vi "sequencerCycleLoops.vi"(6 "kepcoScan":bool, 8 "nOfCycles":i32 format="%0d", 9 "nOfLoops":i32 format="%0d", 11 "Array of Tracks":i32[](array[numeric])=[0, 0, 0, 0, 0, 0, 0, 0, 0, 0, 0, 0, 0, 0, 0, 0, 0, 0, 0, 0, 0, 0, 0, 0, 0, 0, 0, 0, 0, 0, 0, 0, 0, 0, 0, 0, 0, 0, 0, 0, 0, 0, 0, 0, 0, 0, 0, 0, 0, 0, 0, 0, 0, 0, 0, 0, 0, 0, 0, 0, 0, 0, 0, 0, 0, 0, 0, 0, 0]) -> ()   [LabVIEW 2014]
uses:
  <vilib>/rvi/Emulation/niFpgaGetClockAttributes.vi
  <vilib>/rvi/Emulation/niFpgaSctlEmulationGetInTimedLoop.vi
  <vilib>/rvi/Emulation/niFpgaEmulationReportErrorSimple.vi
  sequencerGlobVars.vi
  <vilib>/rvi/Emulation/niFpgaCriticalErrorInLSC.vi
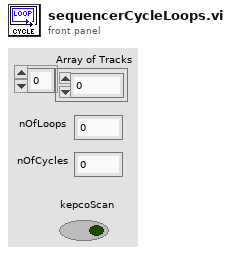
[diagram p1: front panel]
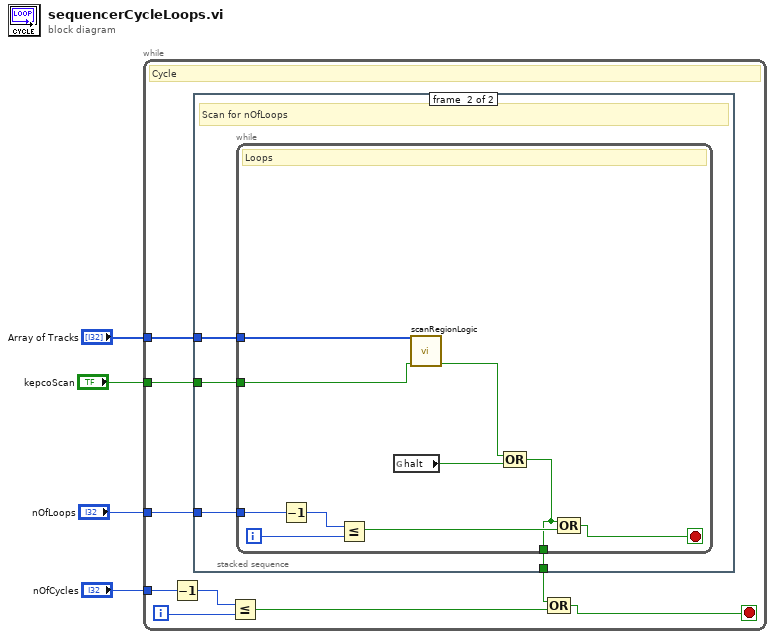
[diagram p0: block diagram]
diagram:
  n1 = while {
    tunnel: "nOfCycles" -> [w12]
    tunnel: "nOfLoops" -> [w10]
    tunnel: "Array of Tracks" -> [w9]
    tunnel: "kepcoScan" -> [w5]
    i -> [w11]
    stop <- w7 stop-if-true
    # "Cycle"
    n2 = Decrement(x=w12) -> (x-1=w13:i32)
    n3 = stacked-sequence {
      tunnel: w10 -> [_ w17]
      tunnel: w9 -> [_ w16]
      tunnel: [_ w15] -> w6
      tunnel: w5 -> [_ w14]
      frame #0 {
        # "measure Offset Voltage"
      }
      frame #1 {
        # "Scan for nOfLoops"
        n4 = while {
          tunnel: w17 -> [w26]
          tunnel: w16 -> [w24]
          tunnel: [w19] -> w15
          tunnel: w14 -> [w18]
          i -> [w25]
          stop <- w20 stop-if-true
          # "Loops"
          n5 = Decrement(x=w26) -> (x-1=w27:i32)
          n6 = Less Or Equal?(x=w27, y=w25) -> (x <= y?=w21:bool)
          n7 = global read "sequencerGlobVars.vi" "halt"() -> (w22:bool)
          n8 = call "scanRegionLogic.vi"("kepcoScan"=w18, "Array of Tracks"=w24) -> ("Error"=w23:bool)  [unwired: 9 in]
          n9 = Compound Arithmetic op=OR(w23, w22) -> (w19:bool)
          n10 = Compound Arithmetic op=OR(w19, w21) -> (w20:bool)
        }
      }
    }
    n11 = Less Or Equal?(x=w13, y=w11) -> (x <= y?=w8:bool)
    n12 = Compound Arithmetic op=OR(w6, w8) -> (w7:bool)
  }
